vi "globalSetUp.vi"(8 "error in (no error)":errorcluster, 11 "testcase-CSMGlobalLog in":refnum<class "testcase-CSMGlobalLog.lvclass">) -> (0 "error out":errorcluster, 3 "testcase-CSMGlobalLog out":refnum<class "testcase-CSMGlobalLog.lvclass">)   [LabVIEW 2017, in "testcase-CSMGlobalLog.lvclass"]
uses:
  testcase-CSMGlobalLog.lvclass
  <vilib>/addons/_JKI Toolkits/VI Tester/TestCase.llb/TestCase.lvclass
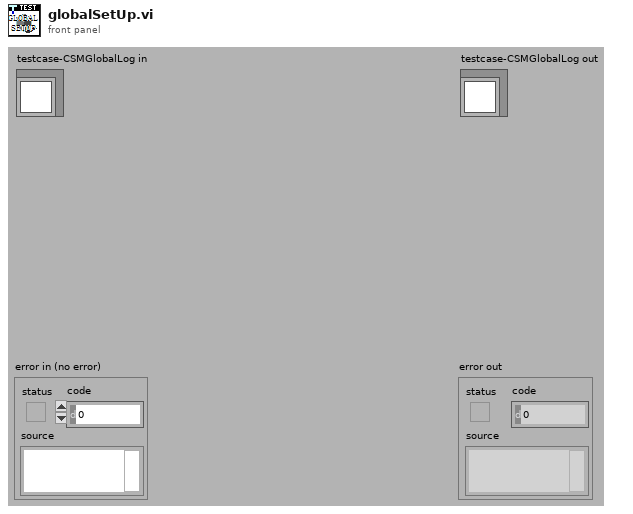
[diagram p1: front panel]
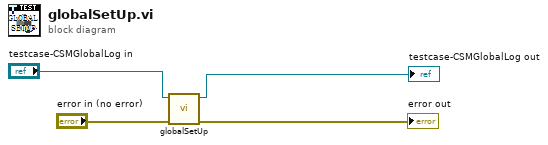
[diagram p0: block diagram]
diagram:
  n1 = call-parent "globalSetUp.vi"("error in (no error)"="error in (no error)", "TestCase in"="testcase-CSMGlobalLog in") -> ("error out"=→"error out":errorcluster, "TestCase out"=→"testcase-CSMGlobalLog out":refnum<class "testcase-CSMGlobalLog.lvclass">)  [unwired: 8 in]
